vi "Test Control.vi"() -> ()   [LabVIEW 2014]
uses:
  Tau.xctl
  <vilib>/Platform/TimedLoop/XDataNode/timing_clust.ctl
  <vilib>/Platform/TimedLoop/XDataNode/nitl_modes.ctl
  <vilib>/Platform/TimedLoop/XDataNode/wakeup.ctl
  <vilib>/Platform/TimedLoop/XDataNode/XDataNode.xnode
  <vilib>/Platform/TimedLoop/XDataNode/XDNodeRunTimeDep.lvlib
panel:
  in  "Stop Button":bool
  out "1D Buffer":cluster{"time":timestamp, "data":sgl[]}(xcontrol)
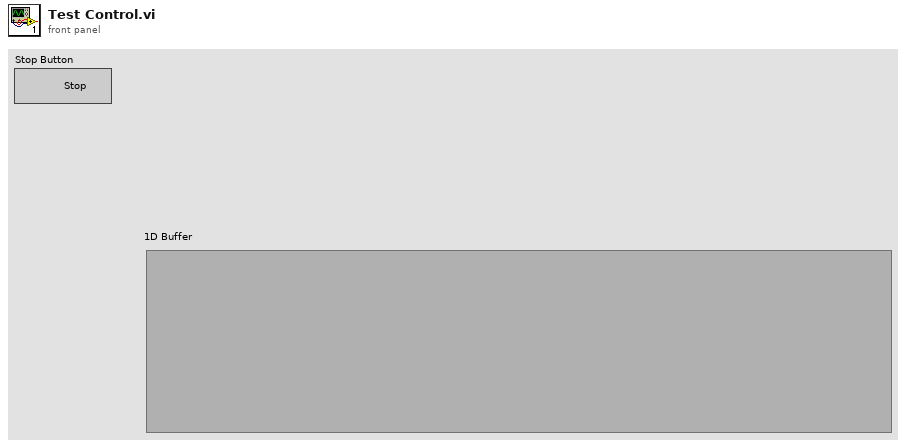
[diagram p1: front panel]
types:
  T1 = cluster{"Name":string, "Line Width":u8, "Line Style":u8, "Color":u32}[]
  T2 = typedef "XDNodeRunTimeDep.lvlib/timing_clust.ctl" = cluster{"Expected End [f-1]":u64, "Actual End [f-1]":u64, "Finished Late? [f-1]":bool, "Expected End [i-1]":u64, "Actual End [i-1]":u64, "Finished Late? [i-1]":bool, "Expected Start [i]":u64, "Actual Start [i]":u64, "Expected Start [f]":u64, "Actual Start [f]":u64, "Source Name":string, "Structure Name":string, "Period":i64, "Deadline":i64, "Offset":i64, "Start":i64, "Priority":i32, "Timeout":i32, "Mode":T3, "Wakeup Reason":T4, "Error":errorcluster, "Source Type":string, "Secondary Source Type":string, "Global End Time":u64, "Global Start Time":u64, "Frame Duration":u64, "Iteration Duration":u64, "Assigned CPU":i32, "I/O Scan Engine Mode":u32}
  T3 = typedef "XDNodeRunTimeDep.lvlib/nitl_modes.ctl" = enum32{"No Change", "Process missed periods, maintain original phase", "Discard missed periods, maintain original phase", "Process missed periods, ignore original phase", "Discard missed periods, ignore original phase"}
  T4 = typedef "XDNodeRunTimeDep.lvlib/wakeup.ctl" = enum32{"Normal", "Aborted", "Asynchronous wakeup", "Timing source error", "Timed loop error", "Timeout"}
  T5 = cluster{"seconds since 1Jan1904":timestamp, dbl[]}
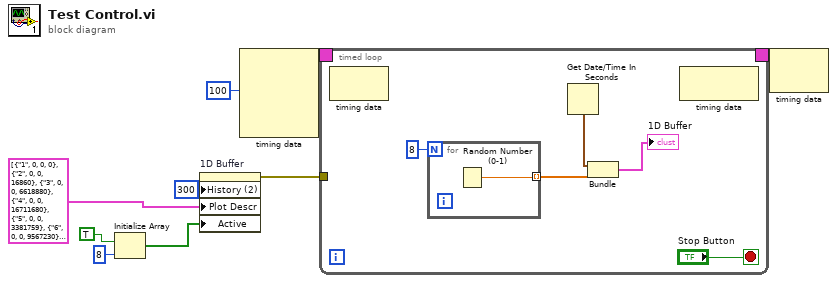
[diagram p0: block diagram]
diagram:
  n1 = Initialize Array(TRUE, 8 ("dimension size")) -> (w2:bool[])
  n2 = property on="1D Buffer" class="1D Buffer (strict)"("History (2)"=u16 300 ("History"), "Plot Descr"=T1 [{"Name"="1", "Line Width"=0, "Line Style"=0, "Color"=0}, {"Name"="2", "Line Width"=0, "Line Style"=0, "Color"=16860}, {"Name"="3", "Line Width"=0, "Line Style"=0, "Color"=6618880}, {"Name"="4", "Line Width"=0, "Line Style"=0, "Color"=16711680}, {"Name"="5", "Line Width"=0, "Line Style"=0, "Color"=3381759}, {"Name"="6", "Line Width"=0, "Line Style"=0, "Color"=9567230}, {"Name"="7", "Line Width"=0, "Line Style"=0, "Color"=12369084}, {"Name"="8", "Line Width"=0, "Line Style"=0, "Color"=1985280}], "Active"=w2) -> (error out=w5:errorcluster)  [unwired: 2 in, 1 out]
  n3 = node-c288(i64 100 ("Period")) -> (w9:T2)  [unwired: 3 in]
  n4 = timed-loop {
    timing: w9 -> [_]
    timing-out: [_] -> w8
    tunnel: w5 -> [_]
    stop <- "Stop Button" stop-if-true
    n5 = node-c288() -> ()  [unwired: 1 in, 1 out]
    n6 = for {
      N: 8 -> [_]
      tunnel: [w17] -> w11 mode=indexing
      n7 = Random Number (0-1)() -> (number: 0 to 1=w17:dbl)
    }
    n8 = Get Date/Time In Seconds() -> (seconds since 1Jan1904=w12:timestamp)
    n9 = Bundle("seconds since 1Jan1904"=w12, w11) -> (→"1D Buffer":T5)  [unwired: 1 in]
    n10 = node-c288() -> ()  [unwired: 1 in, 1 out]
  }
  n11 = node-c288(w8) -> ()  [unwired: 1 out]
